vi "Shooting.vi"(11 "input cluster":T1) -> ()   [LabVIEW 2015]
uses:
  Joystick/ControlsToCommands.ctl
  References/Refnums.vi
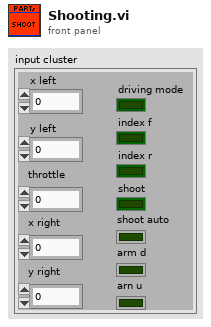
[diagram p1: front panel]
types:
  T1 = typedef "ControlsToCommands.ctl" = cluster{"x left":dbl, "y left":dbl, "throttle":dbl, "x right":dbl, "y right":dbl, "driving mode":bool, "index f":bool, "index r":bool, "shoot":bool, "shoot auto":bool, "arm d":bool, "arn u":bool}
  T2 = typedef "WPI_MotorControlDeviceRef.ctl" = cluster{"DeviceStatus":errorcluster, "Type":T3, "PWM":cluster{"PWM Channel":T4, "DeadBand":T5}, "CAN":cluster{"Device Number":u8, "Control Mode":T6, "Semaphore":T7, "Max Vout":dbl, "TalonSRX Control Mode":T8}, "Invert":bool}
  T3 = typedef "WPI_MotorControlType.ctl" = enum16{"PWM", "CAN", "CANTalonSRX"}
  T4 = typedef "FPGA_DIOPWMChannel.ctl" = enum8{"PWM 0", "PWM 1", "PWM 2", "PWM 3", "PWM 4", "PWM 5", "PWM 6", "PWM 7", "PWM 8", "PWM 9", "PWM MXP 0", "PWM MXP 1", "PWM MXP 2", "PWM MXP 3", "PWM MXP 4", "PWM MXP 5", "PWM MXP 6", "PWM MXP 7", "PWM MXP 8", "PWM MXP 9", "Invalid"}
  T5 = typedef "WPI_PWMDeadband.ctl" = cluster{"Name":string, "maxPositivePwm":i32, "minPositivePwm":i32, "centerPwm":i32, "maxNegativePwm":i32, "minNegativePwm":i32, "angularRange":u16}
  T6 = typedef "WPI_CANJaguar_ControlMode.ctl" = enum8{"Percent VBus", "Current", "Speed", "Position", "Voltage"}
  T7 = typedef "Semaphore RefNum" = refnum<k1>
  T8 = typedef "WPI_CANTalonSRX_APIControlMode.ctl" = enum8{"Percent VBus", "Speed", "Position", "Slave", "Unchanged / Invalid", "Voltage Compensation", "Current", "Motion Profile"}
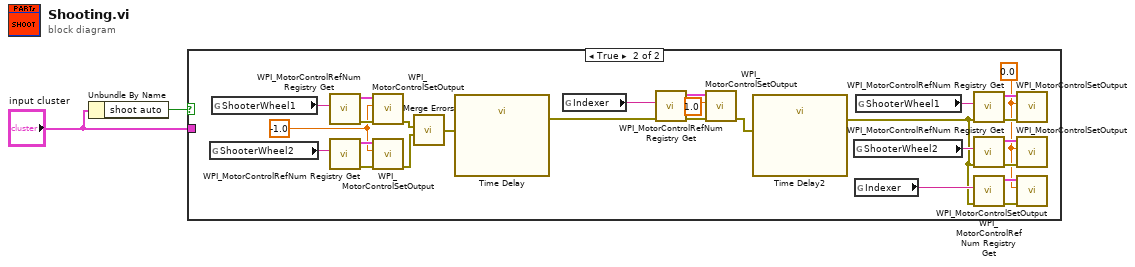
[diagram p0: block diagram]
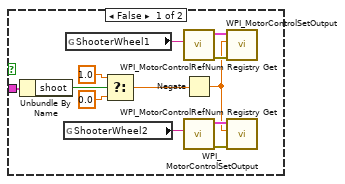
[diagram p2: hidden frame]
diagram:
  n1 = Unbundle By Name("input cluster") -> ("shoot auto"=w2:bool)
  n2 = case shown="True" w2 {
    tunnel: "input cluster" -> [w3 _]
    frame False {
      n3 = Unbundle By Name(w3) -> ("shoot"=w4:bool)
      n4 = global read "Refnums.vi" "ShooterWheel2"() -> (w9:string)
      n5 = global read "Refnums.vi" "ShooterWheel1"() -> (w8:string)
      n6 = Select(t=1.0, s=w4, f=0.0) -> (s? t:f=w14:dbl)
      n7 = call <vilib>:"WPI_MotorControlRefNum Registry Get.vi"("refnum name"=w8) -> ("error out"=w6:errorcluster, "MotorControlDevRef"=w7:T2)  [unwired: 9 in]
      n8 = Negate(x=w14) -> (-x=w5:dbl)
      n9 = call <vilib>:"WPI_MotorControlRefNum Registry Get.vi"("refnum name"=w9) -> ("error out"=w10:errorcluster, "MotorControlDevRef"=w11:T2)  [unwired: 9 in]
      n10 = call <vilib>:"WPI_MotorControlSetOutput.vi"("error in (no error)"=w6, "Output"=w5, "MotorControlDevRef"=w7) -> ()  [unwired: 6 in, 3 out]
      n11 = call <vilib>:"WPI_MotorControlSetOutput.vi"("error in (no error)"=w10, "Output"=w5, "MotorControlDevRef"=w11) -> ()  [unwired: 6 in, 3 out]
    }
    frame True {
      w16 = 0.0
      w35 = -1.0
      n12 = global read "Refnums.vi" "ShooterWheel2"() -> (w39:string)
      n13 = global read "Refnums.vi" "ShooterWheel1"() -> (w38:string)
      n14 = call <vilib>:"WPI_MotorControlRefNum Registry Get.vi"("refnum name"=w38) -> ("error out"=w36:errorcluster, "MotorControlDevRef"=w37:T2)  [unwired: 9 in]
      n15 = call <vilib>:"WPI_MotorControlRefNum Registry Get.vi"("refnum name"=w39) -> ("error out"=w40:errorcluster, "MotorControlDevRef"=w41:T2)  [unwired: 9 in]
      n16 = call <vilib>:"WPI_MotorControlSetOutput.vi"("error in (no error)"=w36, "Output"=w35, "MotorControlDevRef"=w37) -> ("error out"=w34:errorcluster)  [unwired: 6 in, 2 out]
      n17 = call <vilib>:"WPI_MotorControlSetOutput.vi"("error in (no error)"=w40, "Output"=w35, "MotorControlDevRef"=w41) -> ("error out"=w33:errorcluster)  [unwired: 6 in, 2 out]
      n18 = call "Merge Errors.vi"("error in 2"=w33, "error in"=w34) -> ("error out"=w32:errorcluster)  [unwired: 2 in]
      n19 = call "Time Delay"("error in (no error)"=w32) -> ("error out"=w28:errorcluster)  [unwired: 10 in]
      n20 = global read "Refnums.vi" "Indexer"() -> (w29:string)
      n21 = call <vilib>:"WPI_MotorControlRefNum Registry Get.vi"("error in (no error)"=w28, "refnum name"=w29) -> ("error out"=w31:errorcluster, "MotorControlDevRef"=w30:T2)  [unwired: 8 in]
      n22 = call <vilib>:"WPI_MotorControlSetOutput.vi"("error in (no error)"=w31, "Output"=1.0, "MotorControlDevRef"=w30) -> ("error out"=w26:errorcluster)  [unwired: 6 in, 2 out]
      n23 = call "Time Delay2"("error in (no error)"=w26) -> ("error out"=w15:errorcluster)  [unwired: 10 in]
      n24 = global read "Refnums.vi" "ShooterWheel2"() -> (w23:string)
      n25 = global read "Refnums.vi" "Indexer"() -> (w17:string)
      n26 = global read "Refnums.vi" "ShooterWheel1"() -> (w22:string)
      n27 = call <vilib>:"WPI_MotorControlRefNum Registry Get.vi"("error in (no error)"=w15, "refnum name"=w22) -> ("error out"=w20:errorcluster, "MotorControlDevRef"=w21:T2)  [unwired: 8 in]
      n28 = call <vilib>:"WPI_MotorControlRefNum Registry Get.vi"("error in (no error)"=w15, "refnum name"=w23) -> ("error out"=w24:errorcluster, "MotorControlDevRef"=w25:T2)  [unwired: 8 in]
      n29 = call <vilib>:"WPI_MotorControlRefNum Registry Get.vi"("error in (no error)"=w15, "refnum name"=w17) -> ("error out"=w19:errorcluster, "MotorControlDevRef"=w18:T2)  [unwired: 8 in]
      n30 = call <vilib>:"WPI_MotorControlSetOutput.vi"("error in (no error)"=w20, "Output"=w16, "MotorControlDevRef"=w21) -> ()  [unwired: 6 in, 3 out]
      n31 = call <vilib>:"WPI_MotorControlSetOutput.vi"("error in (no error)"=w24, "Output"=w16, "MotorControlDevRef"=w25) -> ()  [unwired: 6 in, 3 out]
      n32 = call <vilib>:"WPI_MotorControlSetOutput.vi"("error in (no error)"=w19, "Output"=w16, "MotorControlDevRef"=w18) -> ()  [unwired: 6 in, 3 out]
    }
  }
